vi "Build.vi"(8 "error in (no error)":errorcluster, 11 "Basic Column Factory in":refnum<class "Basic Column Factory.lvclass">) -> (0 "error out":errorcluster, 2 "Column":refnum<class "Column Interface.lvclass">, 3 "Basic Column Factory out":refnum<class "Basic Column Factory.lvclass">)   [LabVIEW 2020, in "Basic Columns.lvlib" / "Basic Column Factory.lvclass"]
uses:
  Basic Column Factory.lvclass
  Column Interface/Column Interface Class/Column Interface.lvclass
  Basic Column Factory.lvclass/Basic Column Factory.ctl
  Basic Columns/Text Column Class/String Column.lvclass
  C:/Users/User/Desktop/Raman Program/Database OOP/source/Database OOP/Basic Columns/Column Class/Column.lvclass
  Basic Columns/Numeric Column Class/Numeric Column.lvclass
  Basic Columns/Timestamp Column Class/Timestamp Column.lvclass
  Basic Columns/OLE DB Timestamp Class/OLE DB Timestamp.lvclass
  C:/Users/User/Desktop/Raman Program/Database OOP/source/Database OOP/Column Interface/Timestamp Rule Interface/Timestamp Rule Interface.lvclass
  Basic Columns/Timestamp Column Class/Timestamp Column.lvclass/Timestamp Column.ctl
  Basic Columns/Column Class/Column.lvclass
  C:/Users/User/Desktop/Raman Program/Database OOP/source/Database OOP/Column Interface/Column Interface Class/Column Interface.lvclass
  Basic Columns/Basic Column Configuration/Basic Column Configuration.lvclass
  Database Interfaces/Database Interface Class/Database Interface.lvclass
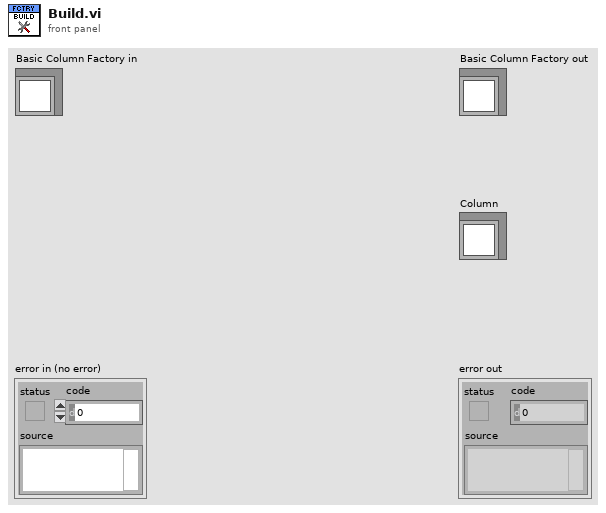
[diagram p1: front panel]
types:
  T1 = typedef "Database Interfaces.lvlib/Database data type.ctl" = enum16{"String", "Long (I32)", "Single (SGL)", "Double (DBL)", "Date/Time", "Binary"}
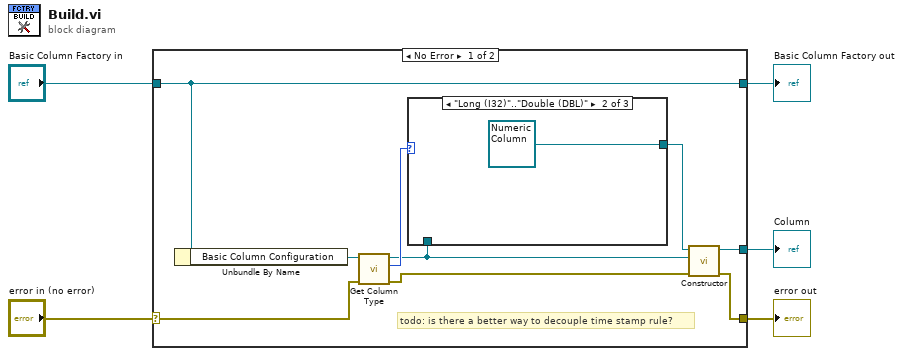
[diagram p0: block diagram]
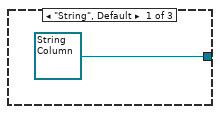
[diagram p2: hidden frame]
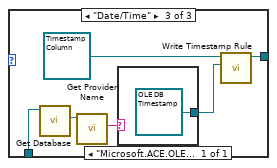
[diagram p3: hidden frame]
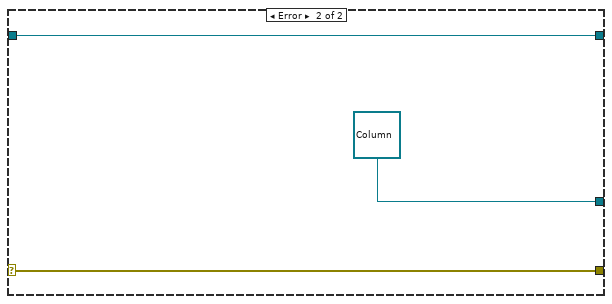
[diagram p4: hidden frame]
diagram:
  n1 = case shown="No Error" "error in (no error)" {
    selector: "error in (no error)" -> [w7 w25]
    tunnel: "Basic Column Factory in" -> [w14 w26]
    tunnel: [w14 w26] -> w3
    tunnel: [w11 w25] -> w2
    tunnel: [w12 refnum<class "Column.lvclass"> refnum ("Column out")] -> w1
    frame No Error {
      # "todo: is there a better way to decouple time stamp rule?"
      n2 = Unbundle By Name(w14) -> ("Basic Column Configuration"=w10:refnum<class "Basic Column Configuration.lvclass">)
      n3 = call-dynamic "Get Column Type.vi"("error in (no error)"=w7, "Basic Column Configuration in"=w10) -> ("error out"=w8:errorcluster, "Column Type"=w9:T1, "Basic Column Configuration out"=w6:refnum<class "Basic Column Configuration.lvclass">)  [unwired: 7 in]
      n4 = case shown="\"Long (I32)\"..\"Double (DBL)\"" w9 {
        tunnel: [refnum<class "String Column.lvclass"> refnum ("Basic Columns.lvlib:String Column.lvclass") refnum<class "Numeric Column.lvclass"> refnum ("Basic Columns.lvlib:Numeric Column.lvclass") w18] -> w13
        tunnel: w6 -> [_ _ w22]
        frame "String", Default {
        }
        frame "Long (I32)".."Double (DBL)" {
        }
        frame "Date/Time" {
          n5 = call-dynamic "Get Database.vi"("Basic Column Configuration in"=w22) -> ("Database"=w21:refnum<class "Database Interface.lvclass">)  [unwired: 8 in, 2 out]
          n6 = call-dynamic "Get Provider Name.vi"("Database Interface in"=w21) -> ("Provider Name"=w20:string)  [unwired: 8 in, 2 out]
          n7 = case shown="\"Microsoft.ACE.OLEDB.16.0\", Default" w20 {
            tunnel: [refnum<class "OLE DB Timestamp.lvclass"> refnum ("Basic Columns.lvlib:OLE DB Timestamp.lvclass")] -> w17
            frame "Microsoft.ACE.OLEDB.16.0", Default {
            }
          }
          n8 = call "Write Timestamp Rule.vi"("Timestamp Rule"=w17, "Timestamp Column in"=refnum<class "Timestamp Column.lvclass"> refnum ("Basic Columns.lvlib:Timestamp Column.lvclass")) -> ("Timestamp Column out"=w18:refnum<class "Timestamp Column.lvclass">)  [unwired: 8 in, 1 out]
        }
      }
      n9 = call-dynamic "Constructor.vi"("error in (no error)"=w8, "Column Configuration"=w6, "Column in"=w13) -> ("error out"=w11:errorcluster, "Column out"=w12:refnum<class "Column.lvclass">)  [unwired: 7 in]
    }
    frame Error {
    }
  }
  "error out" <- w2
  "Basic Column Factory out" <- w3
  "Column" <- w1
